vi "MergeSort.vi"(8 "Sort VI":T1, 11 "ArrayPanelRefs":refnum<data-value>[](array[refnum])) -> (3 "Sorted ArrayPanelRefs":refnum<data-value>[](array[refnum]))   [LabVIEW 2020, in "OOPanel.lvlib" / "ArrayManager.lvclass"]
uses:
  ArrayManager.lvclass
  ArrayPanel/ArrayPanel.lvclass
  Sort VI Type.ctl
  Panel/Panel.lvclass
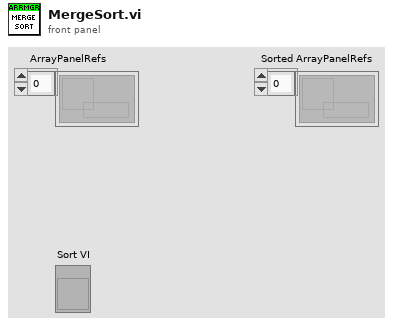
[diagram p1: front panel]
types:
  T1 = typedef "OOPanel.lvlib/ArrayManager.lvclass/Sort VI Type.ctl" = refnum<vi>
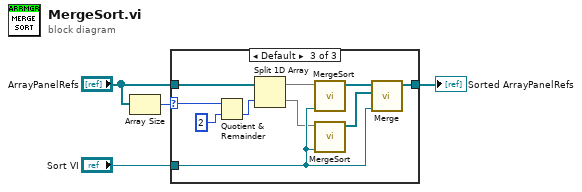
[diagram p0: block diagram]
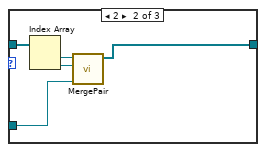
[diagram p3: hidden frame]
diagram:
  n1 = Array Size(array="ArrayPanelRefs") -> (size(s)=w4:i32)
  n2 = case shown="Default" w4 {
    selector: w4 -> [_ _ w18]
    tunnel: "ArrayPanelRefs" -> [w5 w10 w17]
    tunnel: "Sort VI" -> [_ w7 w20]
    tunnel: [w5 w6 w11] -> w1
    frame 0, 1 {
    }
    frame 2 {
      n3 = Index Array(array=w10) -> (element #1=w9:refnum<data-value>, element #2=w8:refnum<data-value>)  [unwired: 2 in]
      n4 = call "MergePair.vi"("Sort VI"=w7, "B"=w8, "A"=w9) -> ("Merged"=w6:refnum<data-value>[])  [unwired: 8 in]
    }
    frame Default {
      n5 = Quotient & Remainder(x=w18, y=2) -> (floor(x/y)=w16:i32)  [unwired: 1 out]
      n6 = Split 1D Array(array=w17, index=w16) -> (first subarray=w14:refnum<data-value>[], second subarray=w15:refnum<data-value>[])
      n7 = call "MergeSort.vi"("Sort VI"=w20, "ArrayPanelRefs"=w14) -> ("Sorted ArrayPanelRefs"=w13:refnum<data-value>[])  [unwired: 9 in]
      n8 = call "MergeSort.vi"("Sort VI"=w20, "ArrayPanelRefs"=w15) -> ("Sorted ArrayPanelRefs"=w12:refnum<data-value>[])  [unwired: 9 in]
      n9 = call "Merge.vi"("Sort VI"=w20, "B"=w12, "A"=w13) -> ("Merged"=w11:refnum<data-value>[])  [unwired: 8 in]
    }
  }
  "Sorted ArrayPanelRefs" <- w1
